vi "U64_to_bool.vi"(3 "N":i32, 4 "N64":u64 format="%b", 5 "IN":bool[](array[boolean])) -> (2 "OUT":bool[](array[boolean]))   [LabVIEW 2019, in "Logik.lvlib"]
uses:
  Logik.lvlib
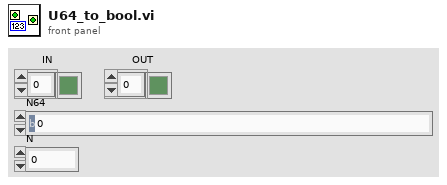
[diagram p1: front panel]
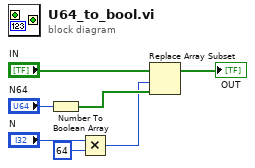
[diagram p0: block diagram]
diagram:
  n1 = Number To Boolean Array(number="N64") -> (Boolean array=w4:bool[])
  n2 = Multiply(x="N", y=64 ("length")) -> (x*y=w3:i32)
  n3 = Replace Array Subset(array="IN", new element=w4, index=w3) -> (→"OUT":bool[])
